vi "list energy peak.vi"() -> (0 "Lines":string[][](array[string]), 1 "Energies Ordered":dbl[](array[numeric]), 2 "List Ordered":string[][](array[string]), 3 "List":string[][](array[string]), 4 "kalpha":string[](array[string]), 5 "Elements":string[][](array[string]))   [LabVIEW 2023]
uses:
  4b7d1e91-fce0-d643-892a-bcd5e833a70f.vi
  <vilib>/Utility/file.llb/Read Delimited Spreadsheet (string).vi
  <vilib>/Utility/Data Type/Get Array Information.vi
  <vilib>/Utility/Data Type/Get Type Information.vi
panel:
  out "appended array":string[][](array[string])
  out "list_peak_energies":string[][](array[string])
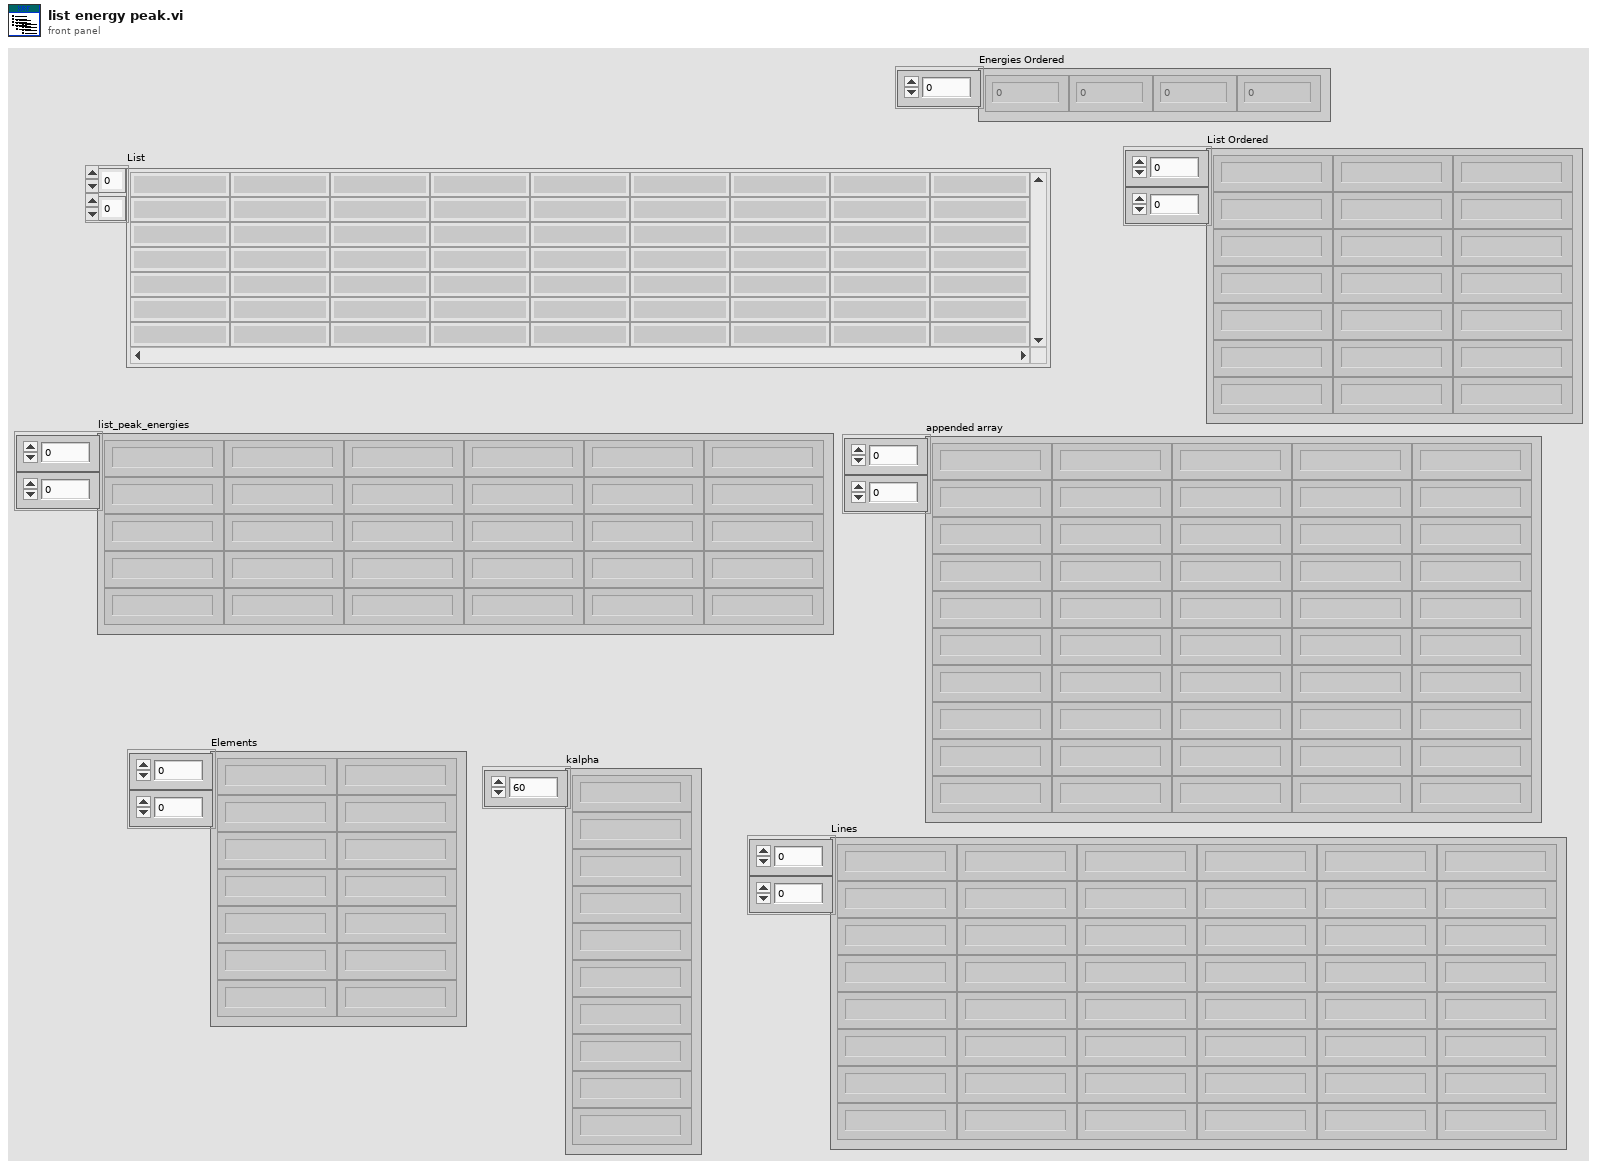
[diagram p1: front panel]
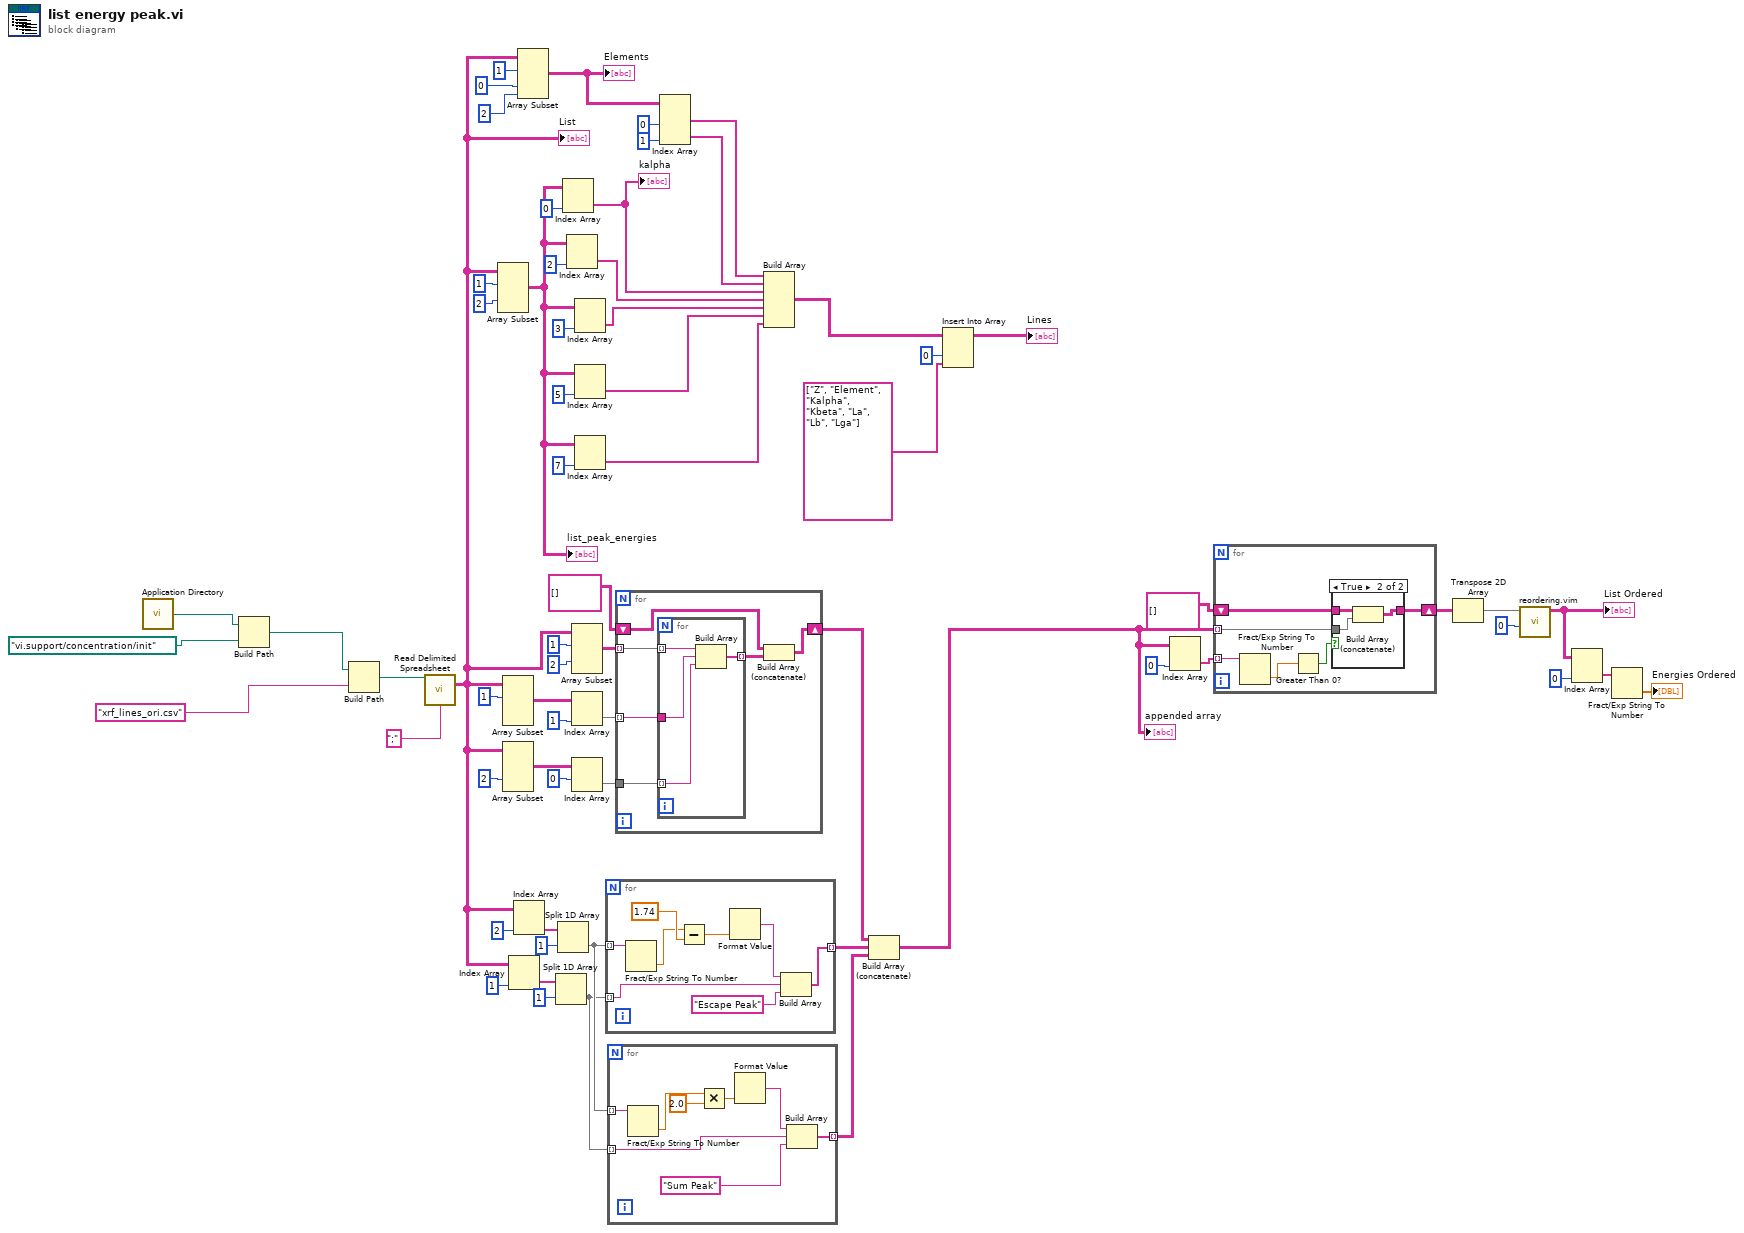
[diagram p0: block diagram]
diagram:
  n1 = call <vilib>:"Application Directory.vi"() -> ("Application Directory"=w3:path)
  n2 = Build Path(base path=w3, name or relative path=path "vi.support/concentration/init") -> (appended path=w1:path)
  n3 = Build Path(base path=w1, name or relative path="xrf_lines_ori.csv") -> (appended path=w65:path)
  n4 = call-poly <vilib>:"Read Delimited Spreadsheet.vi"("file path (dialog if empty)"=w65, "delimiter (\\t)"=";" ("delimiter (\\t)")) -> ("all rows"=w11:string[][])  [unwired: 8 in, 5 out]
  "List" <- w11
  n5 = Array Subset(array=w11, index (row)=1 ("index"), index (col)=2 ("index")) -> (w17:string[][])  [unwired: 2 in]
  "list_peak_energies" <- w17
  n6 = Array Subset(array=w11, index (row)=1 ("index")) -> (w56:string[][])  [unwired: 3 in]
  n7 = Array Subset(array=w11, index (col)=2 ("index")) -> (w58:string[][])  [unwired: 3 in]
  n8 = Index Array(array=w11, index (col)=1 ("disabled index (col)")) -> (element=w37:string[])  [unwired: 1 in]
  n9 = Index Array(array=w11, index (col)=2 ("disabled index (col)")) -> (element=w34:string[])  [unwired: 1 in]
  n10 = Array Subset(array=w11, index (row)=1 ("index"), index (col)=0 ("index"), length (col)=2 ("length")) -> (w8:string[][])  [unwired: 1 in]
  "Elements" <- w8
  n11 = Split 1D Array(array=w37, index=1) -> (second subarray=w32:string[])  [unwired: 1 out]
  n12 = Split 1D Array(array=w34, index=1) -> (second subarray=w33:string[])  [unwired: 1 out]
  n13 = Index Array(array=w17, index (col)=0 ("disabled index (col)")) -> (element=w26:string[])  [unwired: 1 in]
  "kalpha" <- w26
  n14 = Index Array(array=w17, index (col)=2 ("disabled index (col)")) -> (element=w25:string[])  [unwired: 1 in]
  n15 = Array Subset(array=w11, index (row)=1 ("index"), index (col)=2 ("index")) -> (w51:string[][])  [unwired: 2 in]
  n16 = Index Array(array=w56, index (col)=1 ("index (row)")) -> (element=w52:string[])  [unwired: 1 in]
  n17 = Index Array(array=w58, index (row)=0) -> (element=w53:string[])  [unwired: 1 in]
  n18 = Index Array(array=w17, index (col)=3 ("disabled index (col)")) -> (element=w23:string[])  [unwired: 1 in]
  n19 = Index Array(array=w17, index (col)=5 ("disabled index (col)")) -> (element=w21:string[])  [unwired: 1 in]
  n20 = Index Array(array=w17, index (col)=7 ("disabled index (col)")) -> (element=w19:string[])  [unwired: 1 in]
  n21 = for {
    tunnel: w33 -> [w74] mode=indexing
    tunnel: w32 -> [w67] mode=indexing
    tunnel: [w69] -> w31 mode=indexing
    n22 = Fract/Exp String To Number(string=w74) -> (number=w72:dbl)  [unwired: 3 in, 1 out]
    n23 = Subtract(x=w72, y=1.74) -> (x-y=w71:dbl)
    n24 = Format Value(value (0)=w71) -> (output string=w70:string)  [unwired: 2 in]
    n25 = Build Array(w70, w67, "Escape Peak") -> (w69:string[])
  }
  n26 = for {
    tunnel: w33 -> [w82] mode=indexing
    tunnel: w32 -> [w77] mode=indexing
    tunnel: [w75] -> w30 mode=indexing
    n27 = Fract/Exp String To Number(string=w82) -> (number=w80:dbl)  [unwired: 3 in, 1 out]
    n28 = Multiply(x=w80, y=2.0) -> (x*y=w79:dbl)
    n29 = Format Value(value (0)=w79) -> (output string=w78:string)  [unwired: 2 in]
    n30 = Build Array(w78, w77, "Sum Peak") -> (w75:string[])
  }
  n31 = for {
    tunnel: w51 -> [w86] mode=indexing
    tunnel: w53 -> [w88]
    tunnel: w52 -> [w87] mode=indexing
    shift-right: [w83] -> w29
    shift-left: string[][] [] -> [w84]
    n32 = for {
      tunnel: w88 -> [w91] mode=indexing
      tunnel: w87 -> [w92]
      tunnel: w86 -> [w89] mode=indexing
      tunnel: [w90] -> w85 mode=indexing
      n33 = Build Array(w89, w92, w91) -> (w90:string[])
    }
    n34 = Build Array (concatenate)(w84, w85) -> (w83:string[][])
  }
  n35 = Index Array(array=w8, index (col) #1=0 ("disabled index (col)"), index (col) #2=1 ("index (col)")) -> (element #1=w5:string[], element #2=w4:string[])  [unwired: 2 in]
  n36 = Build Array(w5, w4, w26, w25, w23, w21, w19) -> (w16:string[][])
  n37 = Build Array (concatenate)(w29, w31, w30) -> (w28:string[][])
  "appended array" <- w28
  n38 = Insert Into Array(array=w16, index (col)=0 ("disabled index (col)"), new element=string[] ["Z", "Element", "Kalpha", "Kbeta", "La", "Lb", "Lga"]) -> (→"Lines":string[][])  [unwired: 1 in]
  n39 = Index Array(array=w28, index (col)=0 ("disabled index (col)")) -> (element=w48:string[])  [unwired: 1 in]
  n40 = for {
    tunnel: w48 -> [w94] mode=indexing
    tunnel: w28 -> [w97] mode=indexing
    shift-right: [w95] -> w46
    shift-left: string[][] [] -> [w96]
    n41 = Fract/Exp String To Number(string=w94) -> (number=w93:dbl)  [unwired: 3 in, 1 out]
    n42 = Greater Than 0?(x=w93) -> (x > 0?=w98:bool)
    n43 = case shown="True" w98 {
      tunnel: w97 -> [_ w102]
      tunnel: w96 -> [w99 w101]
      tunnel: [w99 w100] -> w95
      frame False {
      }
      frame True {
        n44 = Build Array (concatenate)(w101, w102) -> (w100:string[][])
      }
    }
  }
  n45 = Transpose 2D Array(2D array=w46) -> (transposed array=w45:string[][])
  n46 = call "reordering.vim"("Row to Reorder"=0, "Data In"=w45) -> ("Data Out"=w43:string[][])  [unwired: 8 in, 1 out]
  "List Ordered" <- w43
  n47 = Index Array(array=w43, index (col)=0 ("disabled index (col)")) -> (element=w41:string[])  [unwired: 1 in]
  n48 = Fract/Exp String To Number(string=w41) -> (number=→"Energies Ordered":dbl[])  [unwired: 3 in, 1 out]
